vi "Bin Photon Data in to Images.vi"(0 "# Frames":i32, 3 "Channels":u8[](array[numeric]), 4 "# native bins per user bin (Gate Step/Bin Width)":dbl, 5 "# Pixels Y":i32, 6 "# Gates":i32, 7 "# Pixels X":i32, 8 "Nanotimes":u32[](array[numeric]), 9 "Pixel Durations":u64[](array[numeric]), 10 "New Line Macrotimes":u64[](array[numeric]), 11 "Macrotimes":u64[](array[numeric])) -> (1 "Gate Images":u16[][][](array[numeric]), 2 "Intensity Image":sgl[][](array[numeric]))   [LabVIEW 2021, in "PTU Files.lvlib"]
uses:
  PTU Files.lvlib
  Time/Time.lvlib
panel:
  out "Reshuffling Time (s)":dbl
  out "Binning Time (s)":dbl
  out "Done":bool
  out "Intensity Graph":sgl[][](graph)
  in  "Gate (-1: Intensity)":i32
  in  "Update":bool
  out "size(s)":i32[](array[numeric])
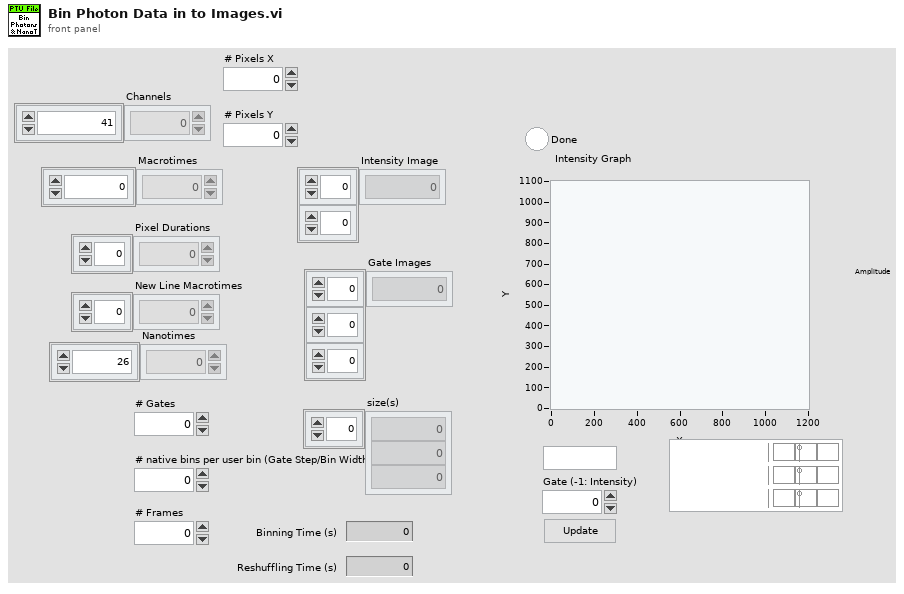
[diagram p1: front panel]
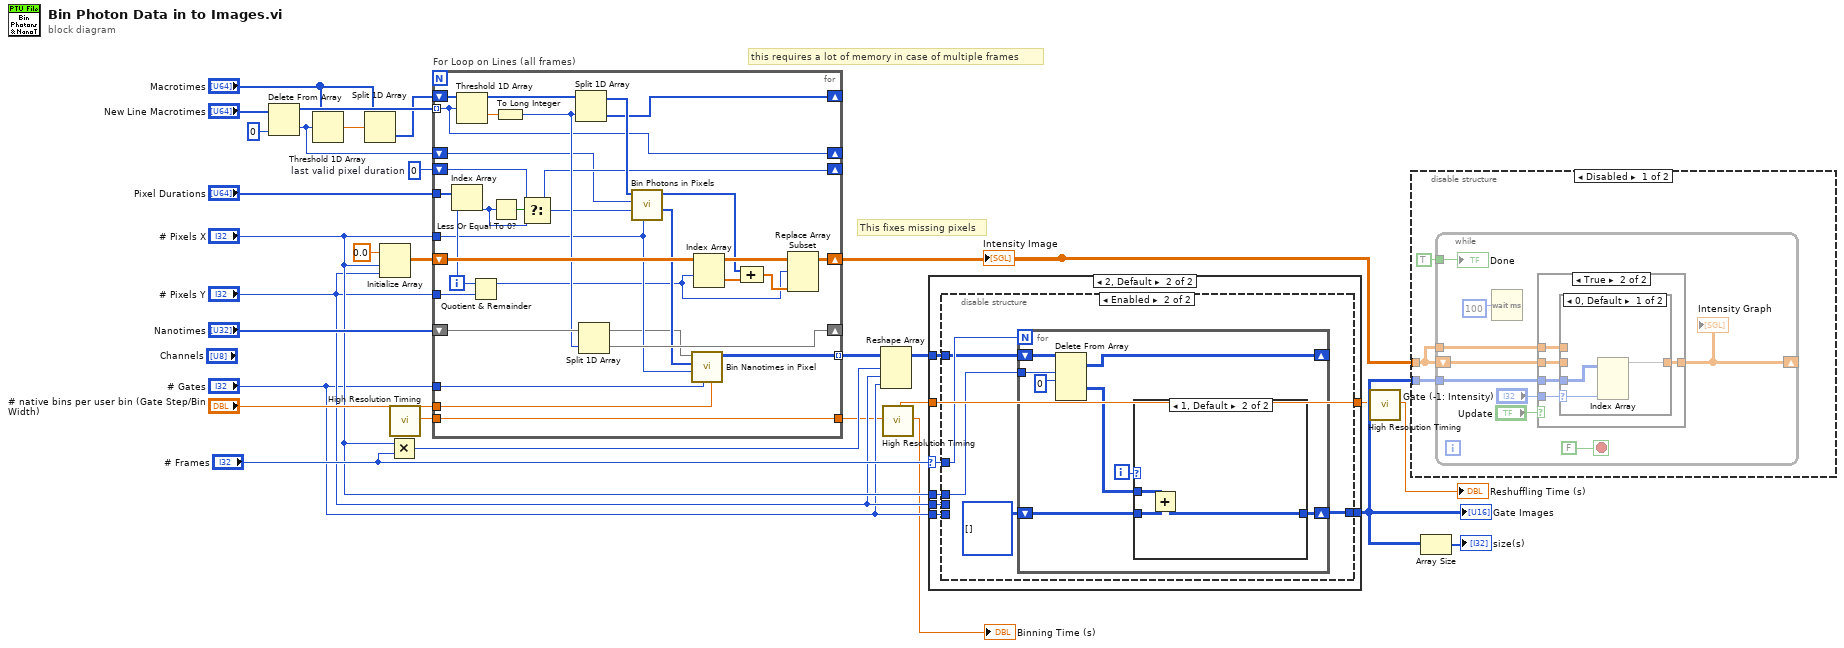
[diagram p0: block diagram]
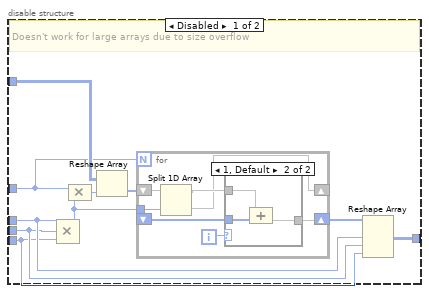
[diagram p6: hidden frame]
diagram:
  w25 = u64 0  # last valid pixel duration
  # "this requires a lot of memory in case of multiple frames"
  # "This fixes missing pixels"
  n1 = Delete From Array(array="New Line Macrotimes", index=0) -> (deleted portion=w16:u64, array with subset deleted=w21:u64[])  [unwired: 1 in]
  n2 = Threshold 1D Array(2:w16, 3:"Macrotimes") -> (0:w18:dbl)  [unwired: 1 in]
  n3 = Split 1D Array(array="Macrotimes", index=w18) -> (second subarray=w17:u64[])  [unwired: 1 out]
  n4 = Initialize Array(sgl 0.0 ("element"), "# Pixels X", "# Pixels Y") -> (w27:sgl[][])
  n5 = Multiply(x="# Pixels X", y="# Frames") -> (x*y=w9:i32)
  n6 = call "High Resolution Timing.vi"() -> ("elapsed (relative) seconds"=w6:dbl)  [unwired: 17 in, 2 out]
  n7 = for "For Loop on Lines (all frames)" {
    tunnel: w21 -> [w35] mode=indexing
    shift-right: [w39] -> _
    shift-left: w17 -> [w42]
    tunnel: "Pixel Durations" -> [w58]
    tunnel: "# Pixels X" -> [w38]
    tunnel: "# Pixels Y" -> [w57]
    shift-right: [w55] -> w13
    shift-left: w27 -> [w56]
    shift-right: [w37] -> _
    shift-left: w25 -> [w50]
    shift-right: [w47] -> _
    shift-left: "Nanotimes" -> [w48]
    tunnel: [w31] -> w15 mode=indexing
    tunnel: "# Gates" -> [w32]
    tunnel: "# native bins per user bin (Gate Step/Bin Width)" -> [w45]
    shift-right: [w35] -> _
    shift-left: w16 -> [w36]
    tunnel: w6 -> [w30]
    tunnel: [w30] -> w5
    i -> [w52]
    n8 = Index Array(array=w58, index=w52) -> (element=w49:u64)
    n9 = Threshold 1D Array(2:w35, 3:w42) -> (0:w43:dbl)  [unwired: 1 in]
    n10 = Quotient & Remainder(x=w52, y=w57) -> (x-y*floor(x/y)=w33:i32)  [unwired: 1 out]
    n11 = Less Or Equal To 0?(x=w49) -> (x <= 0?=w51:bool)
    n12 = To Long Integer(number=w43) -> (32bit integer=w41:i32)
    n13 = Select(t=w50, s=w51, f=w49) -> (s? t:f=w37:u64)
    n14 = Split 1D Array(array=w42, index=w41) -> (first subarray=w40:u64[], second subarray=w39:u64[])
    n15 = Split 1D Array(array=w48, index=w41) -> (first subarray=w34:u32[], second subarray=w47:u32[])
    n16 = call "Bin Photons in Pixels.vi"("# Pixels X"=w38, "Pixel Duration"=w37, "Pixel Start"=w36, "Macrotimes"=w40) -> ("Pixel Boundary Indices"=w44:i32[], "Pixel Values"=w46:i32[])  [unwired: 5 in, 1 out]
    n17 = call "Bin Nanotimes in Pixel.vi"("Nanotime Bin Step"=w45, "# Nanotime Bins"=w32, "# Pixels X"=w38, "Pixel Boundary Indices"=w44, "Nanotimes"=w34) -> ("Gate Lines"=w31:u16[][])  [unwired: 5 in, 1 out]
    n18 = Index Array(array=w56, index (row)=w33) -> (element=w54:sgl[])  [unwired: 1 in]
    n19 = Compound Arithmetic op=ADD(w46, w54) -> (w53:sgl[])
    n20 = Replace Array Subset(array=w56, new element=w53, index (row)=w33) -> (w55:sgl[][])  [unwired: 1 in]
  }
  "Intensity Image" <- w13
  n21 = Reshape Array(w15, w9, "# Pixels Y", "# Gates") -> (w10:u16[][][])
  n22 = call "High Resolution Timing.vi"("relative seconds (NaN)"=w5) -> ("relative seconds"=w3:dbl, "elapsed (relative) seconds"=→"Binning Time (s)":dbl)  [unwired: 16 in, 1 out]
  n23 = case shown="2, Default" "# Frames" {
    selector: "# Frames" -> [_ w66]
    tunnel: w10 -> [w60 w67]
    tunnel: [w60 w65] -> w14
    tunnel: "# Pixels X" -> [_ w64]
    tunnel: "# Pixels Y" -> [_ w63]
    tunnel: "# Gates" -> [_ w62]
    tunnel: w3 -> [w59 w61]
    tunnel: [w59 w61] -> w2
    frame ..1 {
    }
    frame 2, Default {
      n24 = disable-structure shown="Enabled" {
        disable-tunnel: w67 -> [w77 w92]
        disable-tunnel: w66 -> [w74 w93]
        disable-tunnel: [w72 w91] -> w65
        disable-tunnel: w64 -> [w70 w90]
        disable-tunnel: w63 -> [w69 _]
        disable-tunnel: w62 -> [w68 _]
        frame Disabled {
          # "Doesn't work for large arrays due to size overflow"
          n25 = Compound Arithmetic op=MULTIPLY(w70, w69, w68) -> (w71:i32)
          n26 = Compound Arithmetic op=MULTIPLY(w74, w71) -> (w75:i32)
          n27 = Reshape Array(w77, w75) -> (w76:u16[])
          n28 = for {
            N: w74 -> [_]
            shift-right: [w79] -> _
            shift-left: w76 -> [w83]
            shift-right: [w81] -> w73
            shift-left: _ -> [w80]
            tunnel: w71 -> [w78]
            i -> [w84]
            n29 = Split 1D Array(array=w83, index=w78) -> (first subarray=w82:u16[], second subarray=w79:u16[])
            n30 = case shown="1, Default" w84 {
              tunnel: w82 -> [w85 w86]
              tunnel: [w85 w87] -> w81
              tunnel: w80 -> [_ w88]
              frame 0 {
              }
              frame 1, Default {
                n31 = Compound Arithmetic op=ADD(w86, w88) -> (w87:u16[])
              }
            }
          }
          n32 = Reshape Array(w73, w70, w69, w68) -> (w72:u16[][][])
        }
        frame Enabled {
          n33 = for {
            N: w93 -> [_]
            shift-right: [w97] -> _
            shift-left: w92 -> [w101]
            tunnel: w90 -> [w100]
            shift-right: [w96] -> w91
            shift-left: u16[][][] [] ("Gate Lines") -> [w95]
            i -> [w99]
            n34 = Delete From Array(array=w101, length=w100, index (dim 0)=0 ("index (page)")) -> (deleted portion=w98:u16[][][], array with subset deleted=w97:u16[][][])  [unwired: 2 in]
            n35 = case shown="1, Default" w99 {
              tunnel: w98 -> [w102 w105]
              tunnel: [w102 w103] -> w96
              tunnel: w95 -> [_ w104]
              frame 0 {
              }
              frame 1, Default {
                n36 = Add(x=w105, y=w104) -> (x+y=w103:u16[][][])
              }
            }
          }
        }
      }
    }
  }
  "Gate Images" <- w14
  n37 = call "High Resolution Timing.vi"("relative seconds (NaN)"=w2) -> ("elapsed (relative) seconds"=→"Reshuffling Time (s)":dbl)  [unwired: 16 in, 2 out]
  n38 = disable-structure shown="Disabled" {
    disable-tunnel: w14 -> [w108 _]
    disable-tunnel: w13 -> [w107 _]
    frame Disabled {
      n39 = while {
        tunnel: w108 -> [w115]
        shift-right: [w111] -> _
        shift-left: w107 -> [w112]
        tunnel: w107 -> [w113]
        tunnel: TRUE ("Done") -> [w109]
        stop <- FALSE stop-if-true
        n40 = Wait (ms)(milliseconds to wait=u32 100 ("millisecond timer value")) -> ()  [unwired: 1 out]
        n41 = case shown="True" "Update" {
          tunnel: w115 -> [_ w121]
          tunnel: "Gate (-1: Intensity)" -> [_ w123]
          tunnel: w113 -> [_ w122]
          tunnel: [w118 w120] -> w111
          tunnel: w112 -> [w118 w119]
          frame False {
          }
          frame True {
            n42 = case shown="0, Default" w123 {
              selector: w123 -> [w125 _]
              tunnel: w122 -> [_ w127]
              tunnel: w121 -> [w126 _]
              tunnel: [w124 w127] -> w120
              tunnel: w119 -> [_ _]
              frame 0, Default {
                n43 = Index Array(array=w126, index (dim 2)=w125) -> (element=w124:u16[][])  [unwired: 2 in]
              }
              frame ..-1 {
              }
            }
          }
        }
        "Intensity Graph" <- w111
        "Done" <- w109
      }
    }
    frame Enabled {
    }
  }
  n44 = Array Size(array=w14) -> (size(s)=→"size(s)":i32[])
